vi "Latch Solonoid.vi"(11 "Input":bool) -> (3 "Latched":bool)   [LabVIEW 2012]
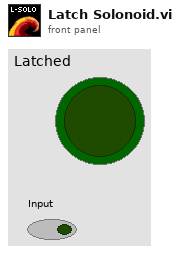
[diagram p1: front panel]
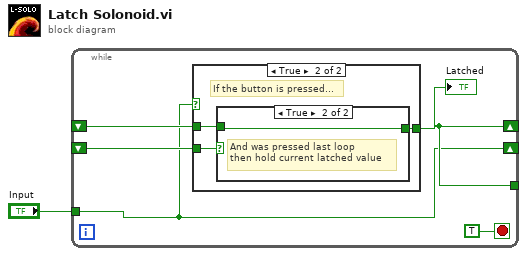
[diagram p0: block diagram]
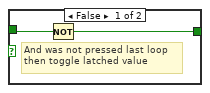
[diagram p3: hidden frame]
diagram:
  n1 = while {
    shift-right: [w2] -> _
    shift-left: _ -> [w6]
    shift-right: [w3] -> _
    shift-left: _ -> [w5]
    tunnel: [w3] -> _
    tunnel: "Input" -> [w2]
    stop <- TRUE stop-if-true
    n2 = case shown="True" w2 {
      tunnel: w6 -> [_ w10]
      tunnel: w5 -> [w7 w9]
      tunnel: [w7 w8] -> w3
      frame False {
        # "then do nothing"
        # "If button is not pressed"
      }
      frame True {
        # "If the button is pressed..."
        n3 = case shown="True" w10 {
          tunnel: w9 -> [w11 w13]
          tunnel: [w12 w13] -> w8
          frame False {
            # "And was not pressed last loop\nthen toggle latched value"
            n4 = Not(x=w11) -> (.not. x?=w12:bool)
          }
          frame True {
            # "And was pressed last loop\nthen hold current latched value"
          }
        }
      }
    }
    "Latched" <- w3
  }
